vi "qSSA.vi"(0 "System no.":i32=1 min=1 max=4 step=1, 2 "Channels to query":string[](array[string]), 3 "All channels?":bool, 4 "Channel identifier?":bool, 5 "error in":errorcluster) -> (14 "Step voltage":dbl[](array[numeric]) format="%.6f", 19 "error out":errorcluster)   [LabVIEW 2020]
doc: "Returns driving voltage amplitude for step mode (step size) of given PiezoWalk channel.\n\nE-755, E-861: If All channels? = TRUE, then Channel identifier? must be FALSE."
panel:
  # "Returns driving voltage amplitude for step mode (step size) of \ngiven PiezoWalk channel."
  # "If all channels: use"
  # "Query"
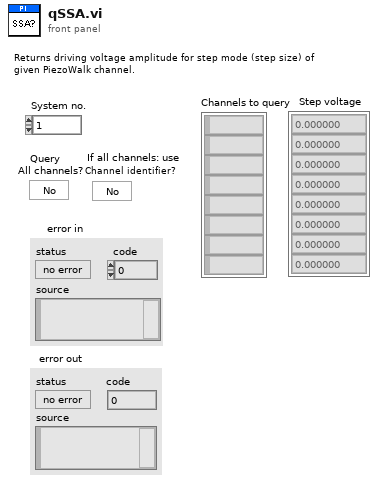
[diagram p1: front panel]
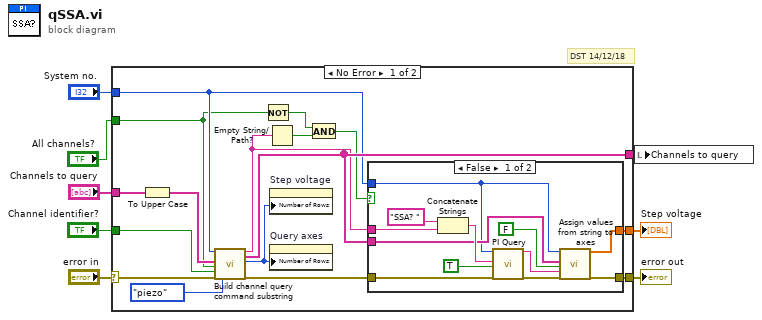
[diagram p0: block diagram]
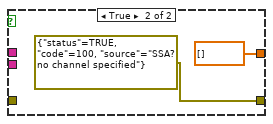
[diagram p2: hidden frame]
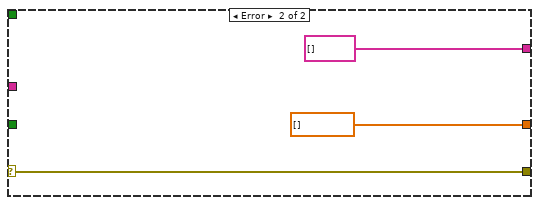
[diagram p3: hidden frame]
diagram:
  # "DST 14/12/18"
  n1 = case shown="No Error" "error in" {
    selector: "error in" -> [w10 w39]
    tunnel: [w24 dbl[] [] ("Values")] -> w8
    tunnel: "Channels to query" -> [w23 _]
    tunnel: [w22 w39] -> w6
    tunnel: "Channel identifier?" -> [w13 _]
    tunnel: "System no." -> [w16 _]
    tunnel: [w18 string[] [] ("Axes to query out")] -> w3
    tunnel: "All channels?" -> [w14 _]
    frame No Error {
      n2 = To Upper Case(1:w23) -> (0:w15:string[])
      n3 = call "Build channel query command substring.vi"("System no."=w16, "Channels to query in"=w15, "Query\nAll channels?"=w14, "For all channels: use\nChannel identifier?"=w13, "error in"=w10, "Channel type"=enum16{"piezo", "sensor"}."piezo") -> ("Command substring"=w12:string, "Channels to query out"=w18:string[], "Number of rows"=w17:u32, "error out"=w19:errorcluster)  [unwired: 1 in, 9 out]
      n4 = Not(x=w14) -> (.not. x?=w21:bool)
      n5 = Empty String/Path?(string/path=w12) -> (empty?=w11:bool)
      n6 = property on="Step voltage" class="Arr (strict)"("Number of Rows"=w17) -> ()  [unwired: 2 in, 2 out]
      n7 = property on="Query axes" class="Arr (strict)"("Number of Rows"=w17) -> ()  [unwired: 2 in, 2 out]
      n8 = And(x=w21, y=w11) -> (x .and. y?=w9:bool)
      n9 = case shown="False" w9 {
        tunnel: [w33 dbl[] [] ("Values")] -> w24
        tunnel: [w32 errorcluster {"status"=TRUE, "code"=100, "source"="SSA? no channel specified"} ("error out")] -> w22
        tunnel: w19 -> [w31 _]
        tunnel: w18 -> [w30 _]
        tunnel: w16 -> [w29 _]
        tunnel: w12 -> [w25 _]
        frame False {
          n10 = Concatenate Strings("SSA? ", w25) -> (w34:string)
          n11 = call "PI Query.vi"("System no."=w29, "String to send"=w34, "Attach termination char.?"=TRUE ("Attach Linefeed?"), "error in"=w31) -> ("String read"=w27:string, "error out"=w26:errorcluster)  [unwired: 3 in, 11 out]
          n12 = call "Assign values from string to axes.vi"("System no."=w29, "Queried axes"=w30, "All axes queried?"=FALSE, "Input String"=w27, "error in"=w26) -> ("Values"=w33:dbl[], "error out"=w32:errorcluster)  [unwired: 4 in, 9 out]
        }
        frame True {
        }
      }
    }
    frame Error {
    }
  }
  "error out" <- w6
  "Step voltage" <- w8
  n13 = local write "Channels to query"(w3) -> ()
